vi "Analysis.Select Raw Data Files.vi"(8 "End":timestamp, 9 "Start":timestamp, 11 "Root Dirs":path[](array[path])) -> (0 "error out":errorcluster, 3 "Data Files":path[](array[path]))   [LabVIEW 2024]
uses:
  Time/Time.DateTime Adjust Action.ctl
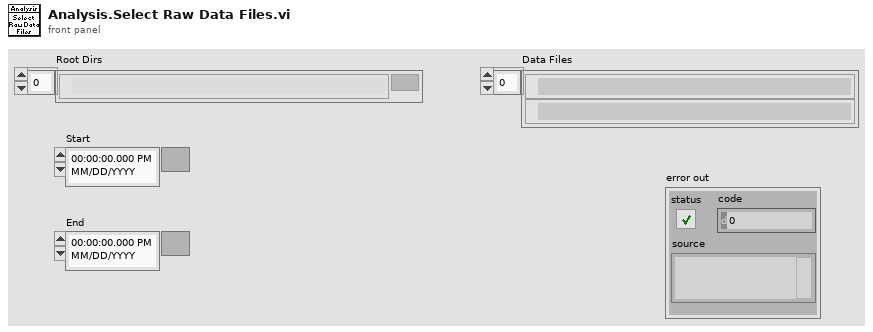
[diagram p1: front panel]
types:
  T1 = typedef "Time.DateTime Adjust Action.ctl" = enum16{"Day Start", "Day End", "Offset Hrs", "UTC to Local", "Local to UTC"}
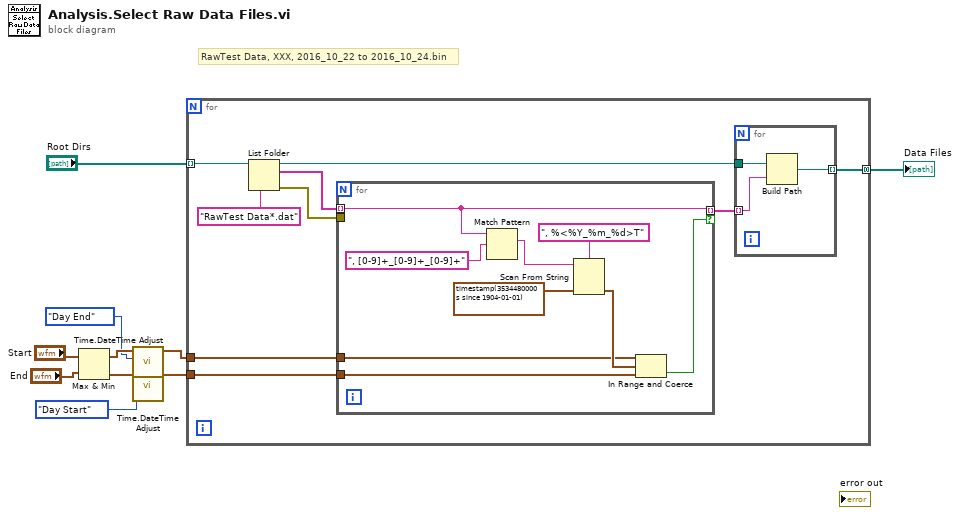
[diagram p0: block diagram]
diagram:
  # "RawTest Data, XXX, 2016_10_22 to 2016_10_24.bin"
  n1 = Max & Min(x="Start", y="End") -> (max(x,y)=w6:timestamp, min(x,y)=w5:timestamp)
  n2 = call "Time.DateTime Adjust.vi"("Action"=Time.DateTime_Adjust_Action."Day End", "Time Stamp"=w6) -> ("Time Stamp Out"=w2:timestamp)  [unwired: 8 in, 1 out]
  n3 = call "Time.DateTime Adjust.vi"("Action"=Time.DateTime_Adjust_Action."Day Start", "Time Stamp"=w5) -> ("Time Stamp Out"=w3:timestamp)  [unwired: 8 in, 1 out]
  n4 = for {
    tunnel: "Root Dirs" -> [w18] mode=indexing
    tunnel: w3 -> [w16]
    tunnel: w2 -> [w15]
    tunnel: [w12] -> w9 mode=concatenating
    n5 = List Folder(path=w18, pattern="RawTest Data*.dat") -> (path out=w13:path, filenames=w19:string[], error out=w11:errorcluster)  [unwired: 2 in, 1 out]
    n6 = for {
      tunnel: w19 -> [w24] mode=indexing
      tunnel: w16 -> [w26]
      tunnel: w15 -> [w25]
      tunnel: [w24] -> w14 mode=indexing if=w23
      tunnel: w11 -> [_]
      n7 = Match Pattern(string=w24, regular expression=", [0-9]+_[0-9]+_[0-9]+" ("time format string (%c)")) -> (match substring=w29:string)  [unwired: 1 in, 3 out]
      n8 = Scan From String(format string=", %<%Y_%m_%d>T", input string=w29, default 1=timestamp(3534480000 s since 1904-01-01) ("default value 1")) -> (output 1=w27:timestamp)  [unwired: 2 in, 3 out]
      n9 = In Range and Coerce(upper limit=w25, x=w27, lower limit=w26) -> (In Range?=w23:bool)  [unwired: 1 out]
    }
    n10 = for {
      tunnel: w14 -> [w21] mode=indexing
      tunnel: w13 -> [w22]
      tunnel: [w20] -> w12 mode=indexing
      n11 = Build Path(base path=w22, name or relative path=w21) -> (appended path=w20:path)
    }
  }
  "Data Files" <- w9
